vi "Set Attributes.vi"(8 "error in (no error)":errorcluster, 11 "Subroutine Dialog in":refnum<class "Subroutine Dialog.lvclass">) -> (0 "error out":errorcluster, 3 "Subroutine Dialog out":refnum<class "Subroutine Dialog.lvclass">)   [LabVIEW 2017, in "Subroutine Dialog.lvclass"]
uses:
  Subroutine Dialog.lvclass
  ITest Executive Builder Dialog/ITest Executive Builder Dialog.lvclass
  <vilib>/gpm_packages/@cs/test-executive/Source/Test Executive/TestExecutive Ref/TestExecutive Ref.lvclass
  788553a5-db11-492c-b925-a5a28d48aafb.vi
  3b1739be-7085-42b1-bd09-05d6d3ee9239.vi
  2205527d-b18a-4e99-a8d6-3d2d98685df2.vi
  C:/Users/jonmc/Documents/Git/Test Executive Builder/Source/Test Executive Builder Dialogs/ITest Executive Builder Dialog/ITest Executive Builder Dialog.lvclass
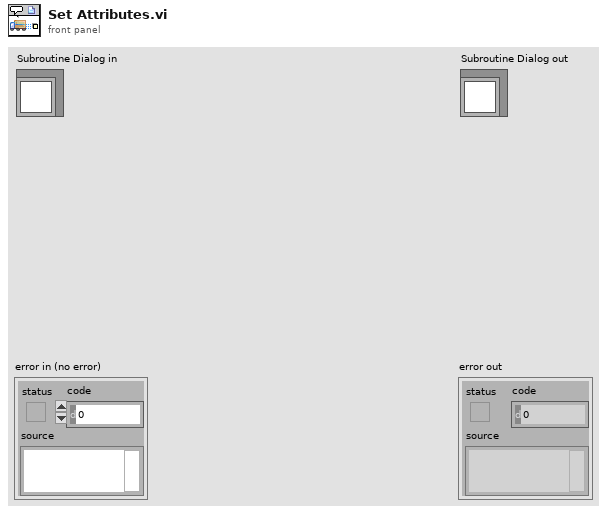
[diagram p1: front panel]
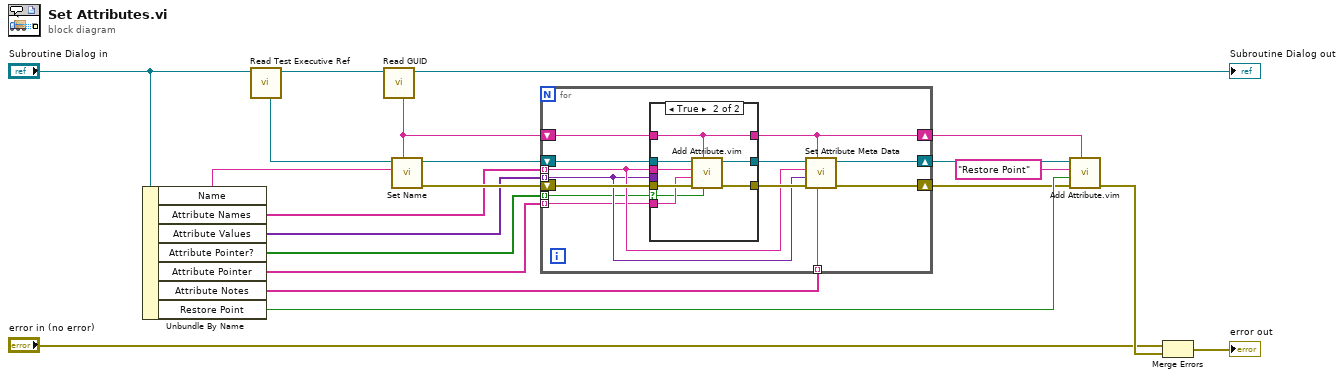
[diagram p0: block diagram]
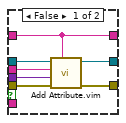
[diagram p2: hidden frame]
diagram:
  n1 = Unbundle By Name("Subroutine Dialog in") -> ("Name"=w19:string, "Attribute Names"=w15:string[], "Attribute Values"=w14:variant[], "Attribute Pointer?"=w6:bool[], "Attribute Pointer"=w5:string[], "Attribute Notes"=w7:string[], "Restore Point"=w13:bool)
  n2 = call "Read Test Executive Ref.vi"("ITest Executive Builder Dialog in"="Subroutine Dialog in") -> ("ITest Executive Builder Dialog out"=w21:refnum<class "Subroutine Dialog.lvclass">, "Test Executive Ref"=w20:refnum<data-value>)  [unwired: 9 in]
  n3 = call "Read GUID.vi"("ITest Executive Builder Dialog in"=w21) -> ("ITest Executive Builder Dialog out"=→"Subroutine Dialog out":refnum<class "Subroutine Dialog.lvclass">, "GUID"=w17:string)  [unwired: 9 in]
  n4 = call <vilib>:"Set Name.vi"("Unique ID"=w17, "Name"=w19, "Test Executive Ref"=w20) -> ("error out"=w16:errorcluster, "Test Executive Ref out"=w18:refnum<data-value>)  [unwired: 7 in]
  n5 = for {
    shift-right: [w31] -> w9
    shift-left: w18 -> [w34]
    shift-right: [w29] -> w8
    shift-left: w16 -> [w33]
    tunnel: w15 -> [w27] mode=indexing
    tunnel: w14 -> [w26] mode=indexing
    shift-right: [w22] -> w10
    shift-left: w17 -> [w25]
    tunnel: w7 -> [w28] mode=indexing
    tunnel: w6 -> [w24] mode=indexing
    tunnel: w5 -> [w23] mode=indexing
    n6 = case shown="True" w24 {
      selector: w24 -> [_ w42]
      tunnel: w34 -> [w41 w49]
      tunnel: w33 -> [w40 w48]
      tunnel: [w39 w47] -> w32
      tunnel: [w38 w46] -> w30
      tunnel: w27 -> [w37 w45]
      tunnel: w26 -> [w36 _]
      tunnel: w25 -> [w35 w44]
      tunnel: w23 -> [_ w43]
      tunnel: [w35 w44] -> w22
      frame False {
        n7 = call "Add Attribute.vim"("ID"=w35, "error in (no error)"=w40, "Attribute"=w36, "Attribute Name"=w37, "Test Executive Ref"=w41) -> ("error out"=w38:errorcluster, "Test Executive Ref out"=w39:refnum<data-value>)  [unwired: 3 in, 2 out]
      }
      frame True {
        n8 = call "Add Attribute.vim"("Pointer?"=w42, "ID"=w44, "error in (no error)"=w48, "Attribute"=w43, "Attribute Name"=w45, "Test Executive Ref"=w49) -> ("error out"=w46:errorcluster, "Test Executive Ref out"=w47:refnum<data-value>)  [unwired: 2 in, 2 out]
      }
    }
    n9 = call <vilib>:"Set Attribute Meta Data.vi"("Meta Data"=w28, "Unique ID"=w22, "error in (no error)"=w30, "Attribute Type"=w26, "Attribute Name"=w27, "Test Executive Ref"=w32) -> ("error out"=w29:errorcluster, "Test Executive Ref out"=w31:refnum<data-value>)  [unwired: 3 in, 1 out]
  }
  n10 = call "Add Attribute.vim"("ID"=w10, "error in (no error)"=w8, "Attribute"=w13, "Attribute Name"="Restore Point", "Test Executive Ref"=w9) -> ("error out"=w11:errorcluster)  [unwired: 3 in, 3 out]
  n11 = Merge Errors("error in (no error)", w11) -> (→"error out":errorcluster)
